vi "sg Set VSB.vi"(7 "symbolCount":i32, 8 "error in (no error)":errorcluster, 9 "symbols":i32, 10 "symbolRate":dbl, 11 "device":i32) -> (0 "error out":errorcluster, 1 "symbols out":i32, 3 "function return":u32(ring))   [LabVIEW 2014, in "VSG25A.lvlib"]
doc: "SG_API sgStatus sgSetVSB(int device, double symbolRate, int *symbols, int symbolCount);"
uses:
  VSG25A.lvlib
  sg_api.dll
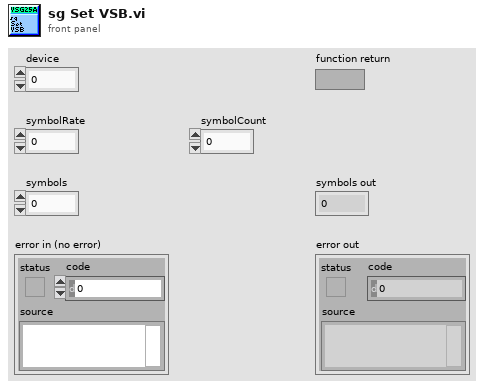
[diagram p1: front panel]
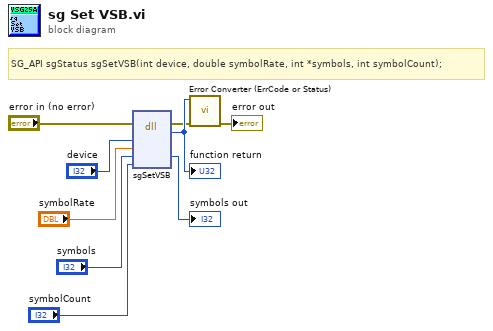
[diagram p0: block diagram]
diagram:
  # "SG_API sgStatus sgSetVSB(int device, double symbolRate, int *symbols, int symbolCount);"
  n1 = dll-call lib="C:/Users/M_LAPTOP/Desktop/Labview/practice/VSG25A/sg_lib/sg_api.*" fn="sgSetVSB"(error in="error in (no error)", "device"="device", "symbolRate"="symbolRate", "symbols"="symbols", "symbolCount"="symbolCount") -> (error out=w2:errorcluster, w9:u32, "symbols"=→"symbols out":i32)  [unwired: 5 in, 1 out]
  "function return" <- w9
  n2 = call "Error Converter (ErrCode or Status).vi"("error in (no error)"=w2, "error code"=w9) -> ("error out"=→"error out":errorcluster)  [unwired: 9 in]
